vi "Module ID.vi"(11 "Data Processor Module in":refnum<class "Data Processor Module.lvclass">) -> (2 "Module ID":string)   [LabVIEW 2020, in "VolatusData.lvlib" / "Data Processor Module.lvclass"]
uses:
  Data Processor Module.lvclass
  Data Processor Module.lvclass/Data Processor Module.ctl
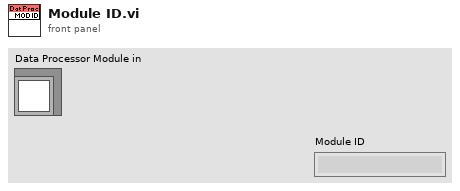
[diagram p1: front panel]
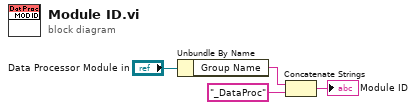
[diagram p0: block diagram]
diagram:
  n1 = Unbundle By Name("Data Processor Module in") -> ("Group Name"=w2:string)
  n2 = Concatenate Strings(w2, "_DataProc" ("string")) -> (→"Module ID":string)
